vi "Temperature Globals.vi"() -> ()   [LabVIEW 2018]
panel:
  out "Last Temp":dbl
  out "Current Temp":dbl
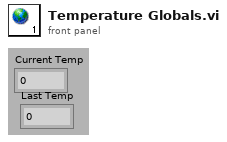
[diagram p1: front panel]
diagram:
